vi "Set Limits on-off.vi"(8 "error in (no error)":errorcluster, 9 "limit lines":bool=TRUE, 10 "limit test":bool=TRUE, 11 "VISA resource name":refnum<visa-resource-name>) -> (0 "error out":errorcluster, 3 "VISA resource name out":refnum<visa-resource-name>)   [LabVIEW 2018, in "Agilent 87XX Series.lvlib"]
doc: "This VI for the HP8753B Network Analyzer is used to turn on and off the limit tests and the limit lines on the instrument display"
uses:
  Agilent 87XX Series.lvlib
panel:
  # "ON\nOFF"
  # "ON\nOFF"
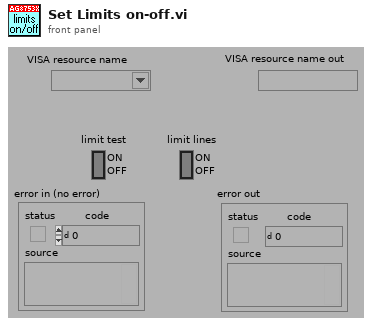
[diagram p1: front panel]
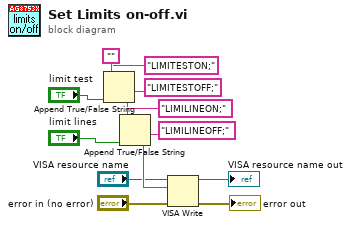
[diagram p0: block diagram]
diagram:
  n1 = Append True/False String(1:"limit test", 2:"LIMITESTOFF;", 3:"LIMITESTON;", 4:"") -> (0:w8:string)
  n2 = Append True/False String(1:"limit lines", 2:"LIMILINEOFF;", 3:"LIMILINEON;", 4:w8) -> (0:w5:string)
  n3 = VISA Write(VISA resource name="VISA resource name", write buffer=w5, error in (no error)="error in (no error)") -> (VISA resource name out=→"VISA resource name out":refnum<visa-resource-name>, error out=→"error out":errorcluster)  [unwired: 1 out]
